vi "UpdateMaxMinTime.vi"(9 "Minimum (msec)":u32=4294967295, 10 "Maximum (msec)":u32, 11 "LastTime (msec)":u32) -> (1 "MinimumOut (msec)":u32=4294967295, 2 "MaximumOut (msec)":u32, 3 "LastTimeOut (msec)":u32)   [LabVIEW 2010]
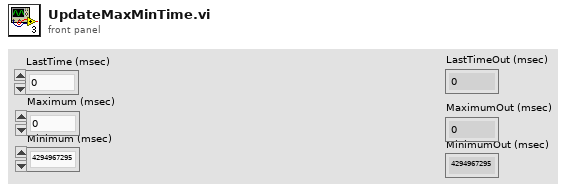
[diagram p1: front panel]
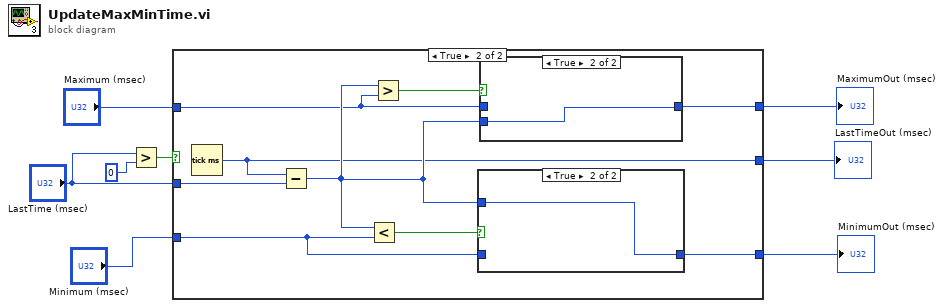
[diagram p0: block diagram]
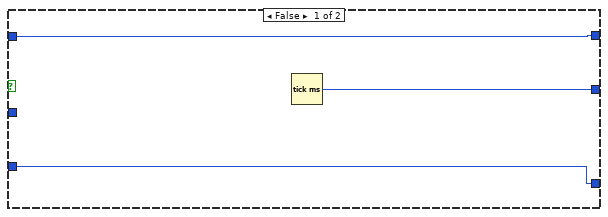
[diagram p2: hidden frame]
diagram:
  n1 = Greater?(x="LastTime (msec)", y=u32 0) -> (0:w3:bool)
  n2 = case shown="True" w3 {
    tunnel: "LastTime (msec)" -> [_ w17]
    tunnel: [w9 w16] -> w8
    tunnel: "Minimum (msec)" -> [w10 w15]
    tunnel: [w10 w14] -> w6
    tunnel: "Maximum (msec)" -> [w11 w13]
    tunnel: [w11 w12] -> w4
    frame False {
      n3 = Tick Count (ms)() -> (millisecond timer value=w9:u32)
    }
    frame True {
      n4 = Tick Count (ms)() -> (millisecond timer value=w16:u32)
      n5 = Subtract(x=w16, y=w17) -> (x-y=w18:u32)
      n6 = Less?(x=w18, y=w15) -> (x < y?=w20:bool)
      n7 = Greater?(x=w18, y=w13) -> (0:w19:bool)
      n8 = case shown="True" w20 {
        tunnel: w18 -> [_ w24]
        tunnel: [w23 w24] -> w14
        tunnel: w15 -> [w23 _]
        frame False {
        }
        frame True {
        }
      }
      n9 = case shown="True" w19 {
        tunnel: w18 -> [_ w22]
        tunnel: [w21 w22] -> w12
        tunnel: w13 -> [w21 _]
        frame False {
        }
        frame True {
        }
      }
    }
  }
  "LastTimeOut (msec)" <- w8
  "MinimumOut (msec)" <- w6
  "MaximumOut (msec)" <- w4
